vi "Add New Line.vi"(8 "error in":errorcluster, 11 "objects":T1) -> (0 "error out":errorcluster, 1 "success":bool, 2 "Line Index":i32)   [LabVIEW 2015, in "TDMS datalogger editor node.lvclass"]
uses:
  TDMS datalogger editor node.lvclass
  <vilib>/NI/DCAF/Tag Editor Core/Table API/Table Manager/object ref.ctl
  <vilib>/NI/DCAF/Tag Editor Core/Configuration Editor/Classes/Engine Parent/Engine Parent Editor Node.lvclass
  <vilib>/NI/DCAF/Tag Editor Core/Configuration Editor/Classes/Module editor node/module editor node.lvclass
  <vilib>/NI/DCAF/Tag Editor Core/Table API/Table Manager/Table Manager.lvclass
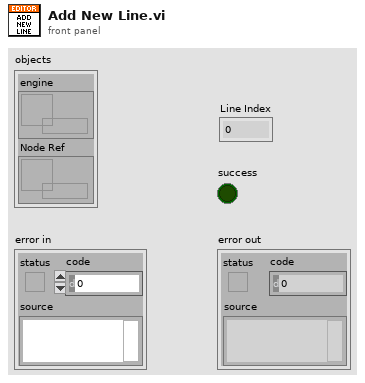
[diagram p1: front panel]
types:
  T1 = typedef "Table Manager.lvlib/Table Manager.lvclass/object ref.ctl" = cluster{"engine":refnum<data-value>, "Node Ref":refnum<data-value>}
  T2 = cluster{"channel":refnum<class "TBM channel.lvclass">}
  T3 = cluster{"Line":cluster{"channel":refnum<class "TBM channel.lvclass">}, "Maps":cluster{"tag name":string, "channel":refnum<class "TBM channel.lvclass">}[]}
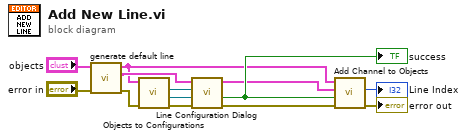
[diagram p0: block diagram]
diagram:
  n1 = call "generate default line.vi"("error in"="error in", "objects in"="objects") -> ("error out"=w11:errorcluster, "Line"=w7:T2, "objects out"=w3:T1)  [unwired: 7 in]
  n2 = call "Objects to Configurations.vi"("error in (no error)"=w11, "Objects in"=w3) -> ("error out"=w10:errorcluster, "engine configuration out"=w9:refnum<class "engine configuration.lvclass">, "TDMS configuration class reference"=w8:refnum<class "TDMS datalogger configuration.lvclass">)  [unwired: 7 in]
  n3 = call "Line Configuration Dialog.vi"("error in"=w10, "engine configuration in"=w9, "TDMS datalogger configuration"=w8, "Line"=w7) -> ("error out"=w6:errorcluster, "success"=w5:bool, "Mappings out"=w4:T3)  [unwired: 4 in, 1 out]
  "success" <- w5
  n4 = call "Add Channel to Objects.vi"("error in"=w6, "Add? (T)"=w5, "Line Item in"=w4, "Objects in"=w3) -> ("error out"=→"error out":errorcluster, "Line Index"=→"Line Index":i32)  [unwired: 6 in]
